vi "FdxCmdRxSAPCreatePortExCvi.vi"(8 "error in":errorcluster, 9 "SapCreateExIn":T1={"PortType"=2, "UdpDst"=0, "IpDst"=0, "VlId"=0, "UdpNumBufMessages"=0, "UdpMaxMessageSize"=0}, 11 "InstrumentHandle_port":u32) -> (0 "error out":errorcluster, 2 "SapHandle":u32, 3 "InstrumentHandle_port":u32)   [LabVIEW 2020, in "AIM664LV.lvlib"]
doc: "Creates a port to receive data from a specified SAP connectionless port. This function can be used only, if receiver is not running. This function assumes that AiFdxCmdRxVLControl was previously called in order to enable a VL for reception. On this VL this function creates an AFDX SAP Rx-port."
uses:
  AIM664LV.lvlib
  AFDX_LibraryAdmin/FdxGlobalDllPath.vi
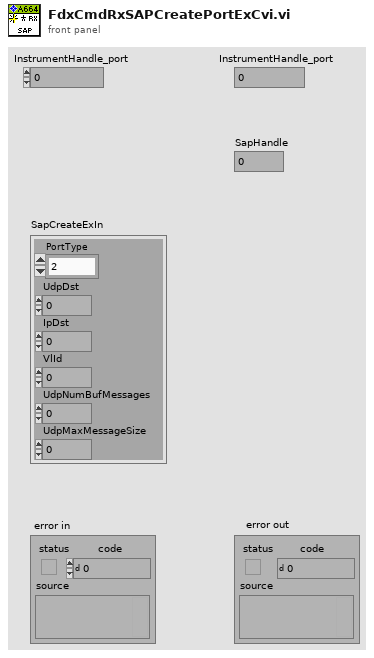
[diagram p1: front panel]
types:
  T1 = cluster{"PortType":u32, "UdpDst":u32, "IpDst":u32, "VlId":u32, "UdpNumBufMessages":u32, "UdpMaxMessageSize":u32}
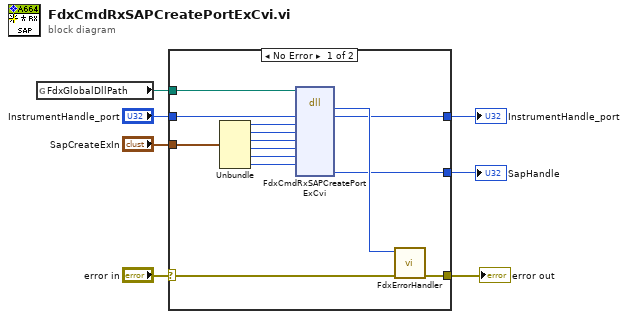
[diagram p0: block diagram]
diagram:
  n1 = global read "FdxGlobalDllPath.vi" "FdxGlobalDllPath"() -> (w5:path)
  n2 = case shown="No Error" "error in" {
    selector: "error in" -> [w20 w23]
    tunnel: [w21 w23] -> w7
    tunnel: w5 -> [w12 _]
    tunnel: [w11 w22] -> w4
    tunnel: "InstrumentHandle_port" -> [w10 w22]
    tunnel: "SapCreateExIn" -> [w9 _]
    tunnel: [w8 _] -> w1
    frame No Error {
      n3 = Unbundle(w9) -> ("PortType"=w18:u32, "UdpDst"=w17:u32, "IpDst"=w16:u32, "VlId"=w15:u32, "UdpNumBufMessages"=w14:u32, "UdpMaxMessageSize"=w13:u32)
      n4 = dll-call lib="aim_fdx.19.dll" fn="FdxCmdRxSAPCreatePortExCvi"(path in=w12, "InstrumentHandle"=w10, "PortType"=w18, "UdpDst"=w17, "IpDst"=w16, "VlId"=w15, "NumBufMessages"=w14, "MaxMessageSize"=w13) -> ("status"=w19:i32, "InstrumentHandle"=w11:u32, "SapHandle"=w8:u32)  [unwired: 8 in, 3 out]
      n5 = call "FdxErrorHandler.vi"("error in"=w20, "AIM Error"=w19) -> ("error out"=w21:errorcluster)  [unwired: 9 in]
    }
    frame Error {
    }
  }
  "error out" <- w7
  "InstrumentHandle_port" <- w4
  "SapHandle" <- w1
